vi "Hormiga_analogRead.vi"(8 "error in (no error)":errorcluster, 10 "Terminal":u8=13, 11 "VISA Refnum in":refnum<visa-resource-name>) -> (0 "error out":errorcluster, 2 "AnalogValue":u16, 3 "VISA Refnum out":refnum<visa-resource-name>)   [LabVIEW 2016]
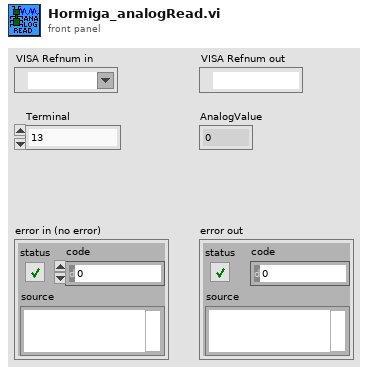
[diagram p1: front panel]
types:
  T1 = enum16{"pinMode", "digitalWrite", "digitalRead", "analogRead", "analogWrite"}
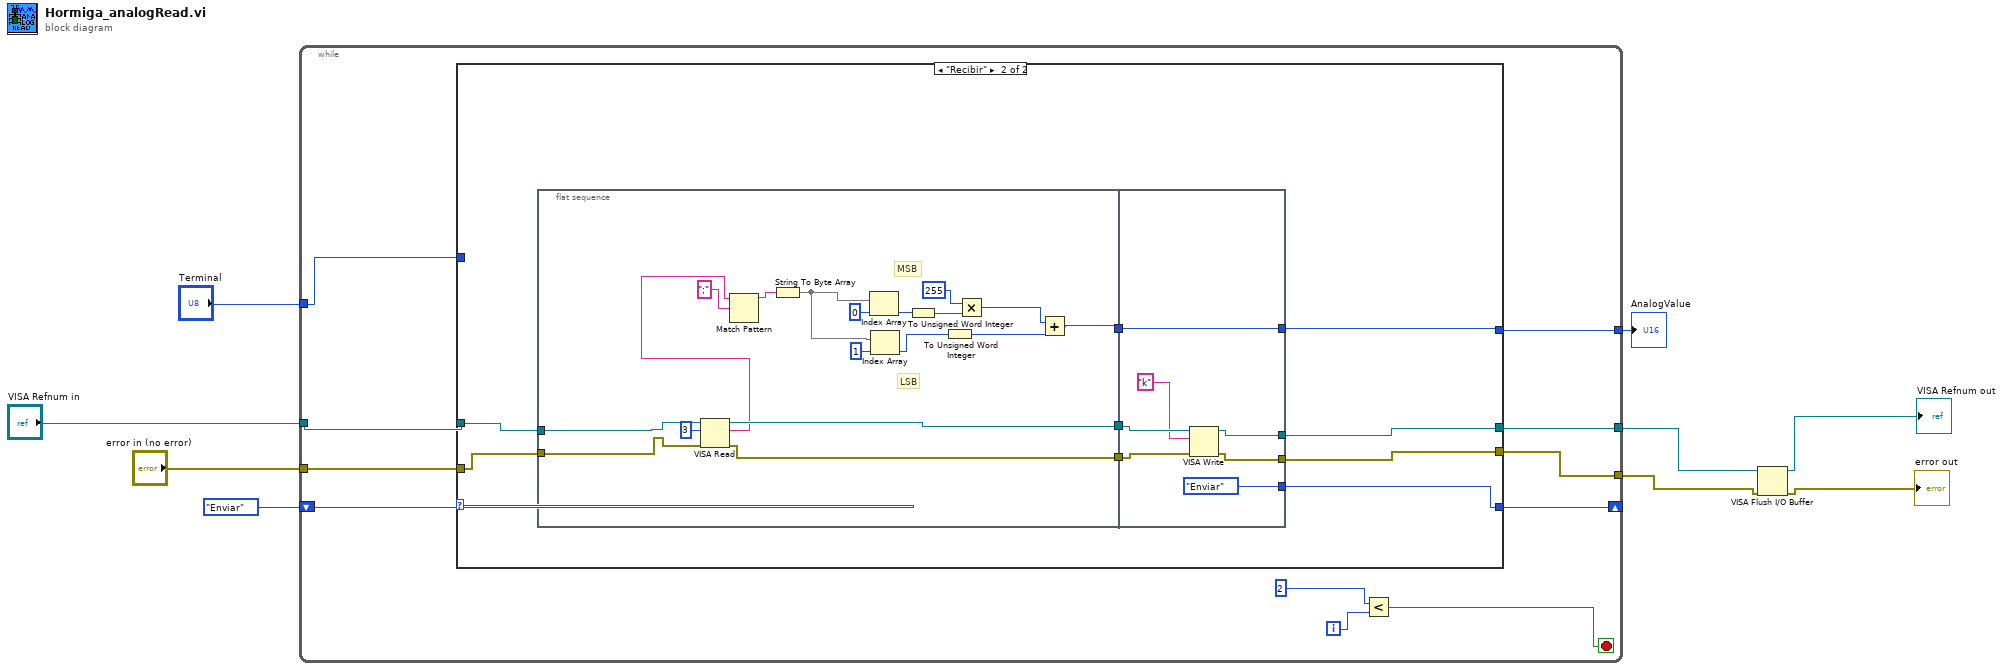
[diagram p0: block diagram]
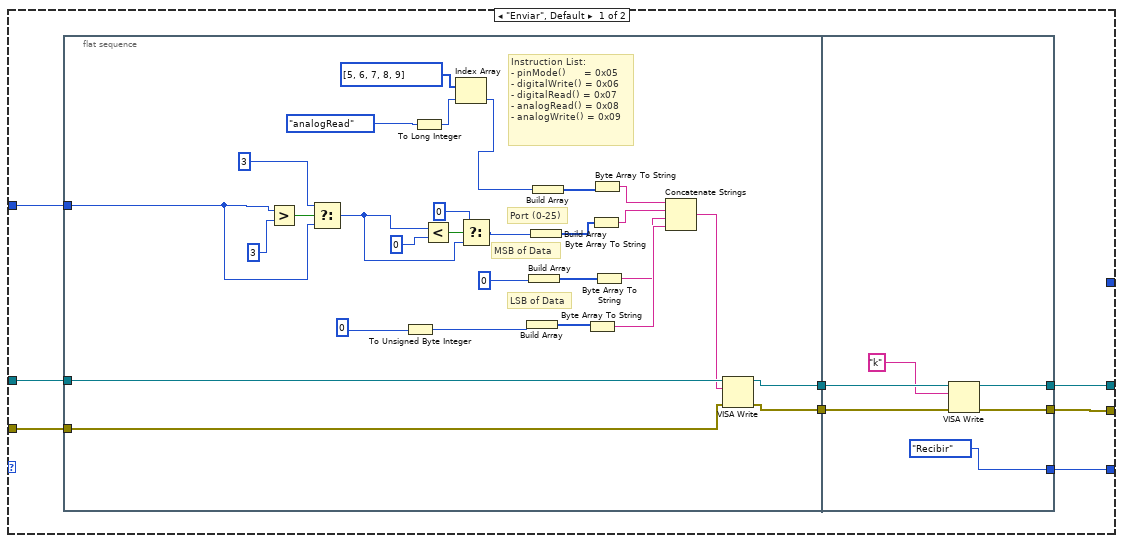
[diagram p2: hidden frame]
diagram:
  n1 = while {
    shift-right: [w15] -> _
    shift-left: enum16{"Enviar", "Recibir"}."Enviar" -> [w20]
    tunnel: "error in (no error)" -> [w19]
    tunnel: "VISA Refnum in" -> [w18]
    tunnel: [w17] -> w1
    tunnel: [w16] -> w2
    tunnel: "Terminal" -> [w11]
    tunnel: [w10] -> w9
    i -> [w13]
    stop <- w14 stop-if-true
    n2 = case shown="\"Recibir\"" w20 {
      tunnel: w19 -> [w28 w72]
      tunnel: w18 -> [w27 w71]
      tunnel: [w24 w68] -> w17
      tunnel: [w23 w67] -> w16
      tunnel: [w22 w66] -> w15
      tunnel: w11 -> [w21 _]
      tunnel: [_ w64] -> w10
      frame "Enviar", Default {
        n3 = flat-sequence {
          tunnel: w28 -> [w57]
          tunnel: w27 -> [w56]
          tunnel: [w55] -> w26
          tunnel: [w54] -> w25
          tunnel: w21 -> [w32]
          tunnel: w26 -> [w63]
          tunnel: w25 -> [w62]
          tunnel: [w60] -> w24
          tunnel: [w59] -> w23
          tunnel: [enum16{"Enviar", "Recibir"}."Recibir"] -> w22
          frame #0 {
            # "Instruction List:\n- pinMode()      = 0x05\n- digitalWrite() = 0x06\n- digitalRead() = 0x07\n- analogRead() = 0x08\n- analogWrite() = 0x09"
            # "LSB of Data"
            # "MSB of Data"
            # "Port (0-25)"
            n4 = Greater?(x=w32, y=u8 3) -> (0:w39:bool)
            n5 = Select(t=u8 3, s=w39, f=w32) -> (s? t:f=w34:u8)
            n6 = To Unsigned Byte Integer(number=u8 0) -> (unsigned 8bit integer=w30:u8)
            n7 = To Long Integer(number=T1."analogRead") -> (32bit integer=w42:i32)
            n8 = Less?(x=w34, y=u8 0) -> (x < y?=w36:bool)
            n9 = Index Array(array=u8[] [5, 6, 7, 8, 9], index=w42) -> (element=w41:u8)
            n10 = Select(t=u8 0, s=w36, f=w34) -> (s? t:f=w33:u8)
            n11 = Build Array(w30) -> (w49:u8[])
            n12 = Build Array(u8 0) -> (w50:u8[])
            n13 = Build Array(w33) -> (w51:u8[])
            n14 = Build Array(w41) -> (w52:u8[])
            n15 = Byte Array To String(unsigned byte array=w49) -> (string=w48:string)
            n16 = Byte Array To String(unsigned byte array=w51) -> (string=w46:string)
            n17 = Byte Array To String(unsigned byte array=w52) -> (string=w45:string)
            n18 = Byte Array To String(unsigned byte array=w50) -> (string=w47:string)
            n19 = Concatenate Strings(w45, w46, w47, w48) -> (w31:string)
            n20 = VISA Write(VISA resource name=w56, write buffer=w31, error in (no error)=w57) -> (VISA resource name out=w54:refnum<visa-resource-name>, error out=w55:errorcluster)  [unwired: 1 out]
          }
          frame #1 {
            n21 = VISA Write(VISA resource name=w62, write buffer="k", error in (no error)=w63) -> (VISA resource name out=w59:refnum<visa-resource-name>, error out=w60:errorcluster)  [unwired: 1 out]
          }
        }
      }
      frame "Recibir" {
        n22 = flat-sequence {
          tunnel: w72 -> [w74]
          tunnel: w71 -> [w75]
          tunnel: [w90] -> w70
          tunnel: [w89] -> w69
          tunnel: [w85] -> w65
          tunnel: w70 -> [w97]
          tunnel: w69 -> [w96]
          tunnel: [w94] -> w68
          tunnel: [w93] -> w67
          tunnel: [enum16{"Enviar", "Recibir"}."Enviar"] -> w66
          tunnel: w65 -> [w91]
          tunnel: [w91] -> w64
          frame #0 {
            # "MSB"
            # "LSB"
            n23 = VISA Read(VISA resource name=w75, byte count=u32 3, error in (no error)=w74) -> (VISA resource name out=w89:refnum<visa-resource-name>, read buffer=w82:string, error out=w90:errorcluster)  [unwired: 1 out]
            n24 = Match Pattern(string=w82, regular expression=";") -> (before substring=w80:string)  [unwired: 1 in, 3 out]
            n25 = String To Byte Array(string=w80) -> (unsigned byte array=w79:u8[])
            n26 = Index Array(array=w79, index=0) -> (element=w78:u8)
            n27 = Index Array(array=w79, index=1) -> (element=w84:u8)
            n28 = To Unsigned Word Integer(number=w78) -> (unsigned 16bit integer=w77:u16)
            n29 = To Unsigned Word Integer(number=w84) -> (unsigned 16bit integer=w83:u16)
            n30 = Multiply(x=u16 255, y=w77) -> (x*y=w76:u16)
            n31 = Add(x=w76, y=w83) -> (x+y=w85:u16)
          }
          frame #1 {
            n32 = VISA Write(VISA resource name=w96, write buffer="k", error in (no error)=w97) -> (VISA resource name out=w93:refnum<visa-resource-name>, error out=w94:errorcluster)  [unwired: 1 out]
          }
        }
      }
    }
    n33 = Less?(x=2, y=w13) -> (x < y?=w14:bool)
  }
  "AnalogValue" <- w9
  n34 = VISA Flush I/O Buffer(VISA resource name=w2, error in (no error)=w1) -> (VISA resource name out=→"VISA Refnum out":refnum<visa-resource-name>, error out=→"error out":errorcluster)  [unwired: 1 in]
